vi "Untitled 5.vi"() -> ()   [LabVIEW 2016]
panel:
  out "array w/ subset deleted":i32[](array[numeric])
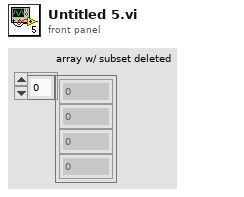
[diagram p1: front panel]
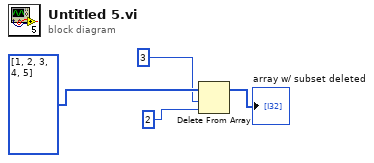
[diagram p0: block diagram]
diagram:
  n1 = Delete From Array(array=i32[] [1, 2, 3, 4, 5], length=3, index=2) -> (array with subset deleted=→"array w/ subset deleted":i32[])  [unwired: 1 out]
